vi "Enqueue Message to all_.vi"(6 "Priority Message? (F)":bool, 8 "error in (no error)":errorcluster, 9 "Message Data":variant, 10 "Message":string, 11 "Message Queues in":T1) -> (0 "error out":errorcluster)   [LabVIEW 2014]
uses:
  All Message Queues.ctl
  Message Cluster.ctl
  Enqueue Message (Single).vi
  Message Queue.lvlib
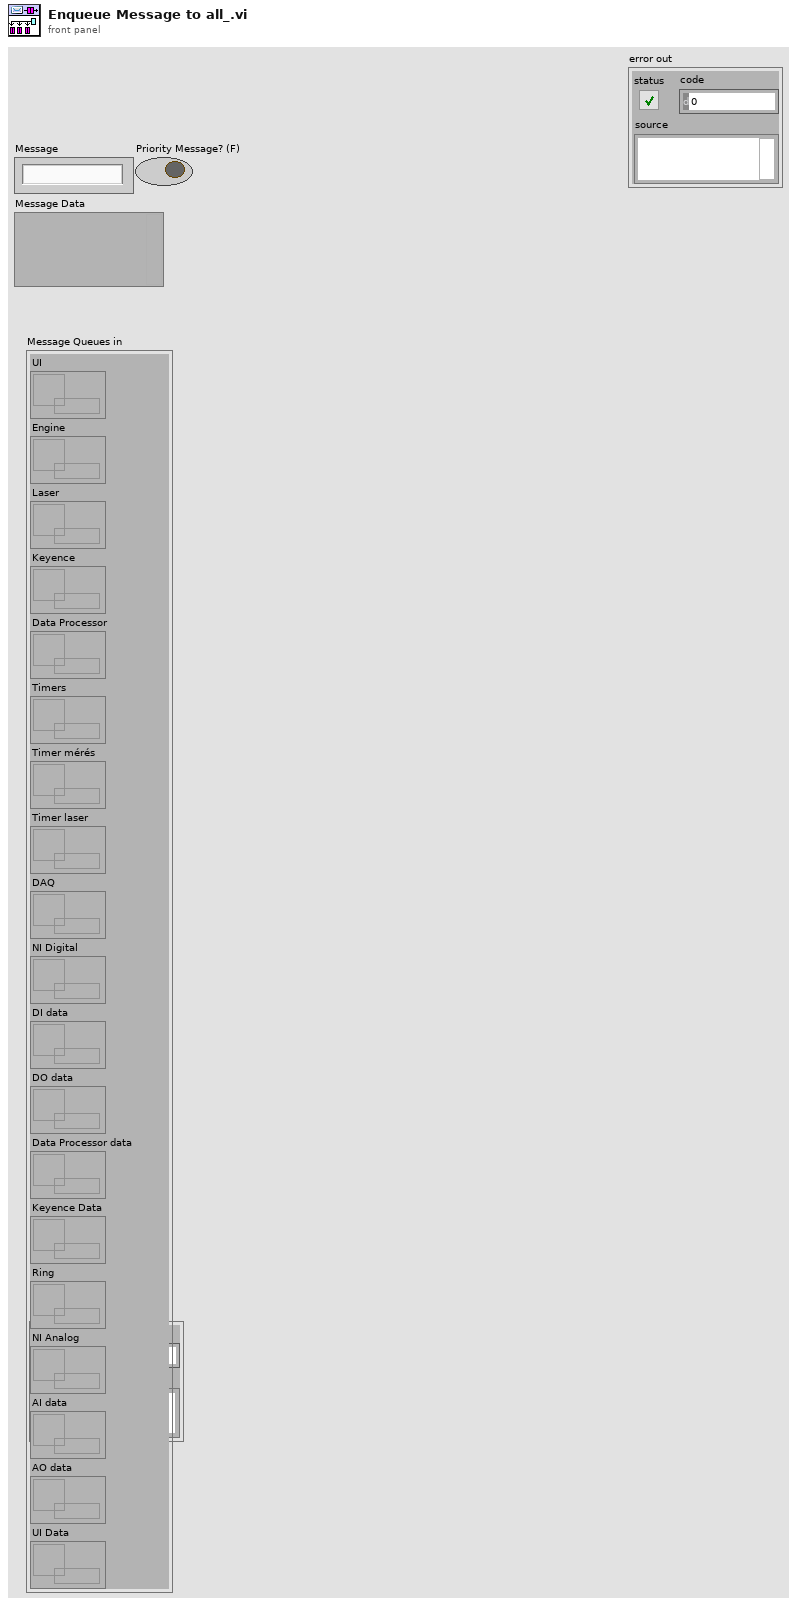
[diagram p1: front panel]
types:
  T1 = typedef "Message Queue.lvlib/All Message Queues.ctl" = cluster{"UI":refnum<queue>, "Engine":refnum<queue>, "Laser":refnum<queue>, "Keyence":refnum<queue>, "Data Processor":refnum<queue>, "Timers":refnum<queue>, "Timer mérés":refnum<queue>, "Timer laser":refnum<queue>, "DAQ":refnum<queue>, "NI Digital":refnum<queue>, "DI data":refnum<queue>, "DO data":refnum<queue>, "Data Processor data":refnum<queue>, "Keyence Data":refnum<queue>, "Ring":refnum<queue>, "NI Analog":refnum<queue>, "AI data":refnum<queue>, "AO data":refnum<queue>, "UI Data":refnum<queue>}
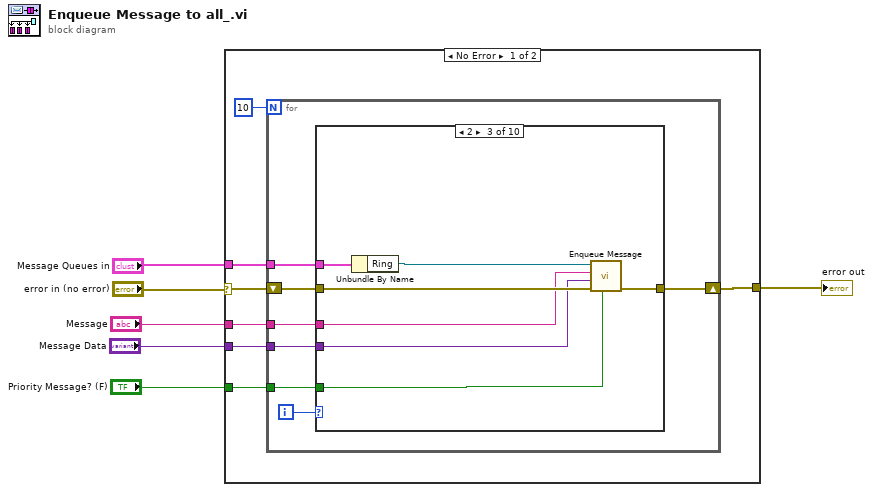
[diagram p0: block diagram]
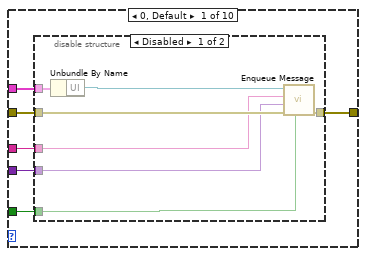
[diagram p2: hidden frame]
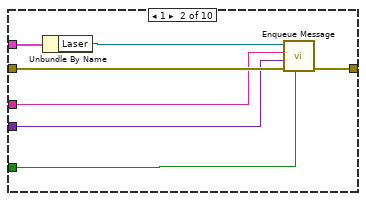
[diagram p4: hidden frame]
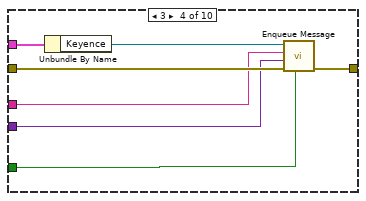
[diagram p5: hidden frame]
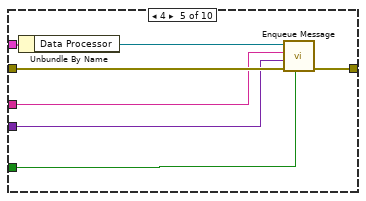
[diagram p6: hidden frame]
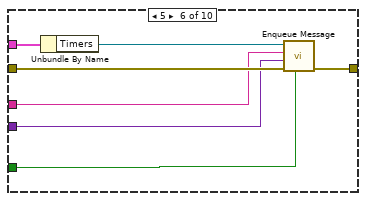
[diagram p7: hidden frame]
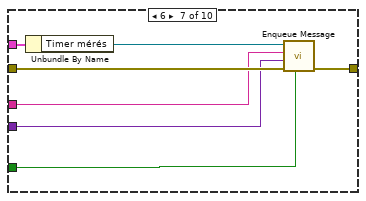
[diagram p8: hidden frame]
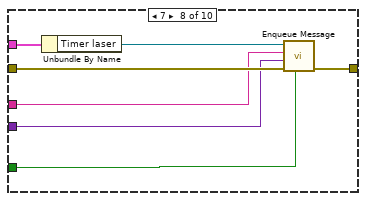
[diagram p9: hidden frame]
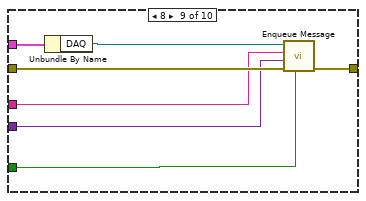
[diagram p10: hidden frame]
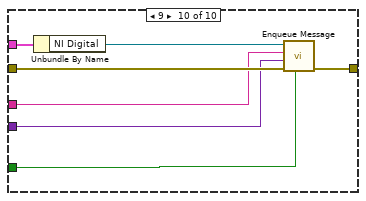
[diagram p11: hidden frame]
diagram:
  n1 = case shown="No Error" "error in (no error)" {
    selector: "error in (no error)" -> [w13 w98]
    tunnel: "Message Queues in" -> [w10 _]
    tunnel: [w11 w98] -> w4
    tunnel: "Priority Message? (F)" -> [w9 _]
    tunnel: "Message Data" -> [w8 _]
    tunnel: "Message" -> [w7 _]
    frame No Error {
      n2 = for {
        N: 10 -> [_]
        shift-right: [w20] -> w11
        shift-left: w13 -> [w19]
        tunnel: w10 -> [w17]
        tunnel: w9 -> [w16]
        tunnel: w8 -> [w15]
        tunnel: w7 -> [w14]
        i -> [w18]
        n3 = case shown="2" w18 {
          tunnel: w19 -> [w25 w39 w46 w53 w60 w67 w74 w81 w88 w95]
          tunnel: w17 -> [w26 w41 w48 w55 w62 w69 w76 w83 w90 w97]
          tunnel: [w24 w38 w45 w52 w59 w66 w73 w80 w87 w94] -> w20
          tunnel: w16 -> [w23 w37 w44 w51 w58 w65 w72 w79 w86 w93]
          tunnel: w15 -> [w22 w36 w43 w50 w57 w64 w71 w78 w85 w92]
          tunnel: w14 -> [w21 w35 w42 w49 w56 w63 w70 w77 w84 w91]
          frame 0, Default {
            n4 = disable-structure shown="Disabled" {
              disable-tunnel: w26 -> [w33 _]
              disable-tunnel: w25 -> [w31 w34]
              disable-tunnel: [w30 w34] -> w24
              disable-tunnel: w23 -> [w29 _]
              disable-tunnel: w22 -> [w28 _]
              disable-tunnel: w21 -> [w27 _]
              frame Disabled {
                n5 = Unbundle By Name(w33) -> ("UI"=w32:refnum<queue>)
                n6 = call-poly "Enqueue Message.vi"("Priority Message? (F)"=w29, "error in (no error)"=w31, "Message Data"=w28, "Message"=w27, "Message Queue"=w32) -> ("error out"=w30:errorcluster)  [unwired: 5 in, 1 out]
              }
              frame Enabled {
              }
            }
          }
          frame 1 {
            n7 = Unbundle By Name(w41) -> ("Laser"=w40:refnum<queue>)
            n8 = call-poly "Enqueue Message.vi"("Priority Message? (F)"=w37, "error in (no error)"=w39, "Message Data"=w36, "Message"=w35, "Message Queue"=w40) -> ("error out"=w38:errorcluster)  [unwired: 5 in, 1 out]
          }
          frame 2 {
            n9 = Unbundle By Name(w48) -> ("Ring"=w47:refnum<queue>)
            n10 = call-poly "Enqueue Message.vi"("Priority Message? (F)"=w44, "error in (no error)"=w46, "Message Data"=w43, "Message"=w42, "Message Queue"=w47) -> ("error out"=w45:errorcluster)  [unwired: 5 in, 1 out]
          }
          frame 3 {
            n11 = Unbundle By Name(w55) -> ("Keyence"=w54:refnum<queue>)
            n12 = call-poly "Enqueue Message.vi"("Priority Message? (F)"=w51, "error in (no error)"=w53, "Message Data"=w50, "Message"=w49, "Message Queue"=w54) -> ("error out"=w52:errorcluster)  [unwired: 5 in, 1 out]
          }
          frame 4 {
            n13 = Unbundle By Name(w62) -> ("Data Processor"=w61:refnum<queue>)
            n14 = call-poly "Enqueue Message.vi"("Priority Message? (F)"=w58, "error in (no error)"=w60, "Message Data"=w57, "Message"=w56, "Message Queue"=w61) -> ("error out"=w59:errorcluster)  [unwired: 5 in, 1 out]
          }
          frame 5 {
            n15 = Unbundle By Name(w69) -> ("Timers"=w68:refnum<queue>)
            n16 = call-poly "Enqueue Message.vi"("Priority Message? (F)"=w65, "error in (no error)"=w67, "Message Data"=w64, "Message"=w63, "Message Queue"=w68) -> ("error out"=w66:errorcluster)  [unwired: 5 in, 1 out]
          }
          frame 6 {
            n17 = Unbundle By Name(w76) -> ("Timer mérés"=w75:refnum<queue>)
            n18 = call-poly "Enqueue Message.vi"("Priority Message? (F)"=w72, "error in (no error)"=w74, "Message Data"=w71, "Message"=w70, "Message Queue"=w75) -> ("error out"=w73:errorcluster)  [unwired: 5 in, 1 out]
          }
          frame 7 {
            n19 = Unbundle By Name(w83) -> ("Timer laser"=w82:refnum<queue>)
            n20 = call-poly "Enqueue Message.vi"("Priority Message? (F)"=w79, "error in (no error)"=w81, "Message Data"=w78, "Message"=w77, "Message Queue"=w82) -> ("error out"=w80:errorcluster)  [unwired: 5 in, 1 out]
          }
          frame 8 {
            n21 = Unbundle By Name(w90) -> ("DAQ"=w89:refnum<queue>)
            n22 = call-poly "Enqueue Message.vi"("Priority Message? (F)"=w86, "error in (no error)"=w88, "Message Data"=w85, "Message"=w84, "Message Queue"=w89) -> ("error out"=w87:errorcluster)  [unwired: 5 in, 1 out]
          }
          frame 9 {
            n23 = Unbundle By Name(w97) -> ("NI Digital"=w96:refnum<queue>)
            n24 = call-poly "Enqueue Message.vi"("Priority Message? (F)"=w93, "error in (no error)"=w95, "Message Data"=w92, "Message"=w91, "Message Queue"=w96) -> ("error out"=w94:errorcluster)  [unwired: 5 in, 1 out]
          }
        }
      }
    }
    frame Error {
    }
  }
  "error out" <- w4
